vi "waterTank.vi"() -> ()   [LabVIEW 2018]
panel:
  out "HOT \nWATER LEVEL":u8(slide) scale=0.0..150.0
  in  "SET TEMPERATURE":dbl(knob) scale=20.0..105.0
  out "GEYSER ON":bool
  in  "GEYSER\nSWITCH":bool
  out "TEMPERATURE":dbl(knob) scale=20.0..105.0
  in  "HOT WATER PUMP":dbl(slide) scale=0.0..150.0
  out "HOT WATER TANK":dbl(slide) scale=0.0..150.0
  out "WATER\n LEVEL":dbl(slide) scale=0.0..500.0
  in  "TANK MOTOR SWITCH":bool
  out "ALARM":bool
  in  "Stop Alarm":bool
  out "PUMP ON":bool
  in  "MAX":dbl(slide) scale=0.0..500.0
  in  "MIN":dbl(slide) scale=0.0..500.0
  in  "MAIN TANK":dbl(slide) scale=0.0..500.0
  out "TANK":dbl(slide) scale=0.0..500.0
  # "WATER LEVEL CONTROL SYSTEM"
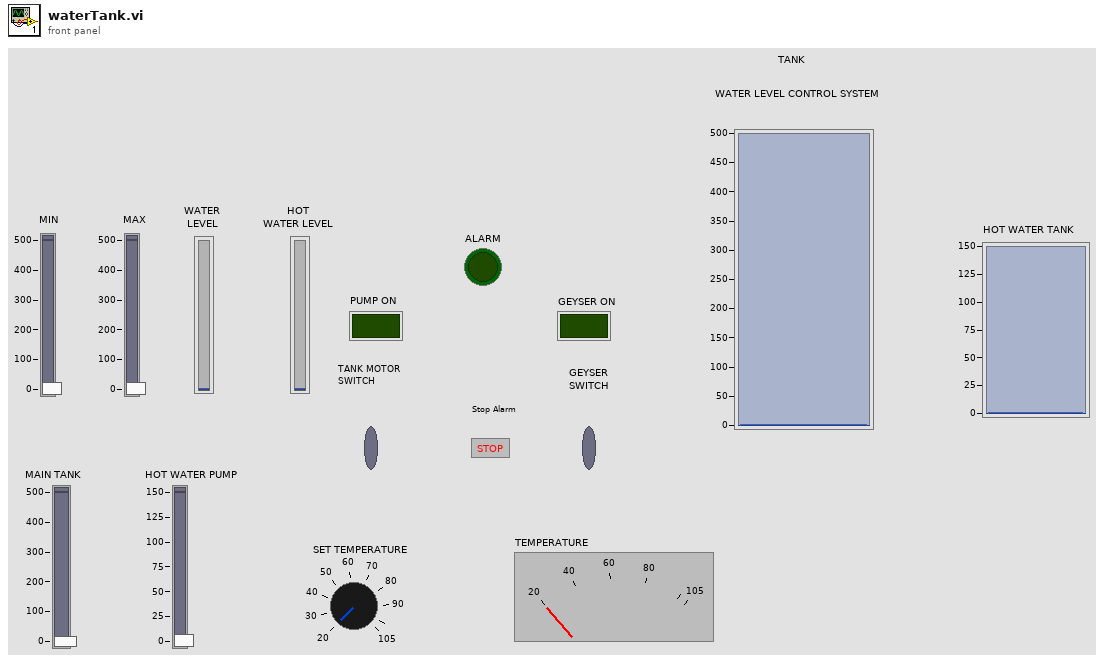
[diagram p1: front panel]
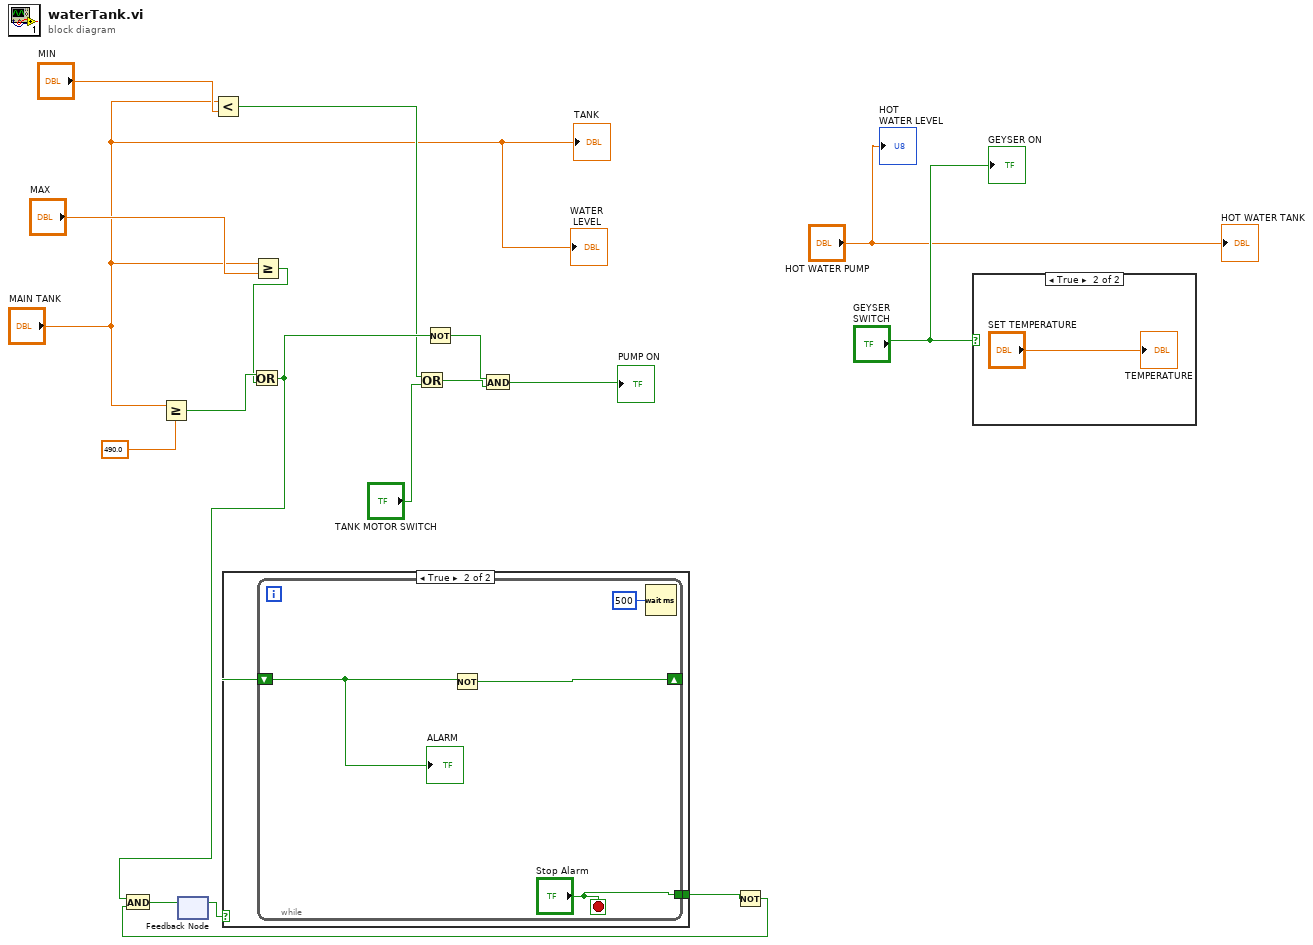
[diagram p0: block diagram]
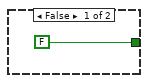
[diagram p3: hidden frame]
diagram:
  n1 = Greater Or Equal?(x="MAIN TANK", y=490.0) -> (x >= y?=w16:bool)
  n2 = feedback #1() -> (w11:bool)  [unwired: 1 in]
  n3 = Less?(x="MAIN TANK", y="MIN") -> (x < y?=w7:bool)
  n4 = case shown="True" w11 {
    selector: w11 -> [_ w21]
    tunnel: [FALSE w20] -> w10
    frame False {
    }
    frame True {
      n5 = while {
        shift-right: [w25] -> _
        shift-left: w21 -> [w22]
        tunnel: ["Stop Alarm"] -> w20
        stop <- "Stop Alarm" stop-if-true
        n6 = Not(x=w22) -> (.not. x?=w25:bool)
        n7 = Wait (ms)(milliseconds to wait=u32 500) -> ()  [unwired: 1 out]
        "ALARM" <- w22
      }
    }
  }
  n8 = Greater Or Equal?(x="MAIN TANK", y="MAX") -> (x >= y?=w4:bool)
  n9 = Or(x=w16, y=w4) -> (x .or. y?=w8:bool)
  n10 = Or(x=w7, y="TANK MOTOR SWITCH") -> (x .or. y?=w5:bool)
  n11 = Not(x=w8) -> (.not. x?=w14:bool)
  n12 = And(x=w14, y=w5) -> (x .and. y?=→"PUMP ON":bool)
  n13 = Not(x=w10) -> (.not. x?=w9:bool)
  n14 = And(x=w8, y=w9) -> (x .and. y?=w12:bool)
  n15 = feedback-in #1(w12) -> ()
  n16 = case shown="True" "GEYSER\nSWITCH" {
    frame False {
    }
    frame True {
      "TEMPERATURE" <- "SET TEMPERATURE"
    }
  }
  "TANK" <- "MAIN TANK"
  "WATER\n LEVEL" <- "MAIN TANK"
  "HOT WATER TANK" <- "HOT WATER PUMP"
  "GEYSER ON" <- "GEYSER\nSWITCH"
  "HOT \nWATER LEVEL" <- "HOT WATER PUMP"
